vi "Mandelbrot.vi"() -> ()   [LabVIEW 2011]
doc: "This VI will create a mandelbrot fractal image. You can modify the colors by changing the map in the color map section. In addition, you can also modify the depth and color scheme by changing the iteration maximum (currently set to 50)."
uses:
  <vilib>/Utility/miscctls.llb/LVBoundsTypeDef.ctl
  <vilib>/Analysis/1siggen.llb/Ramp Pattern by Samples.vi
  <vilib>/gmath/interp.llb/Create Mesh Grid (2D) (x,y arrays).vi
  <vilib>/Analysis/NI_AALBase.lvlib
  <vilib>/gmath/NI_Gmath.lvlib
panel:
  out "Create picture name":string
  out "Zoom":dbl
  out "Min":cdb
  out "Max":cdb
  in  "Picture Folder":path
  in  "Save Button":bool
  in  "Iterations":u32=400
  in  "Resolution":u32=1000
  out "Horizontal Graduated Bar":dbl(slide)=0.999 scale=0.0..1.0
  in  "Reset":bool
  in  "Redraw":bool
  in  "stop":bool
  in  "Im_min":dbl=-2.0
  in  "Im_max":dbl=2.0
  in  "Re_min":dbl=-2.0
  in  "Re_max":dbl=2.0
  out "Intensity Graph":u32[][](graph)
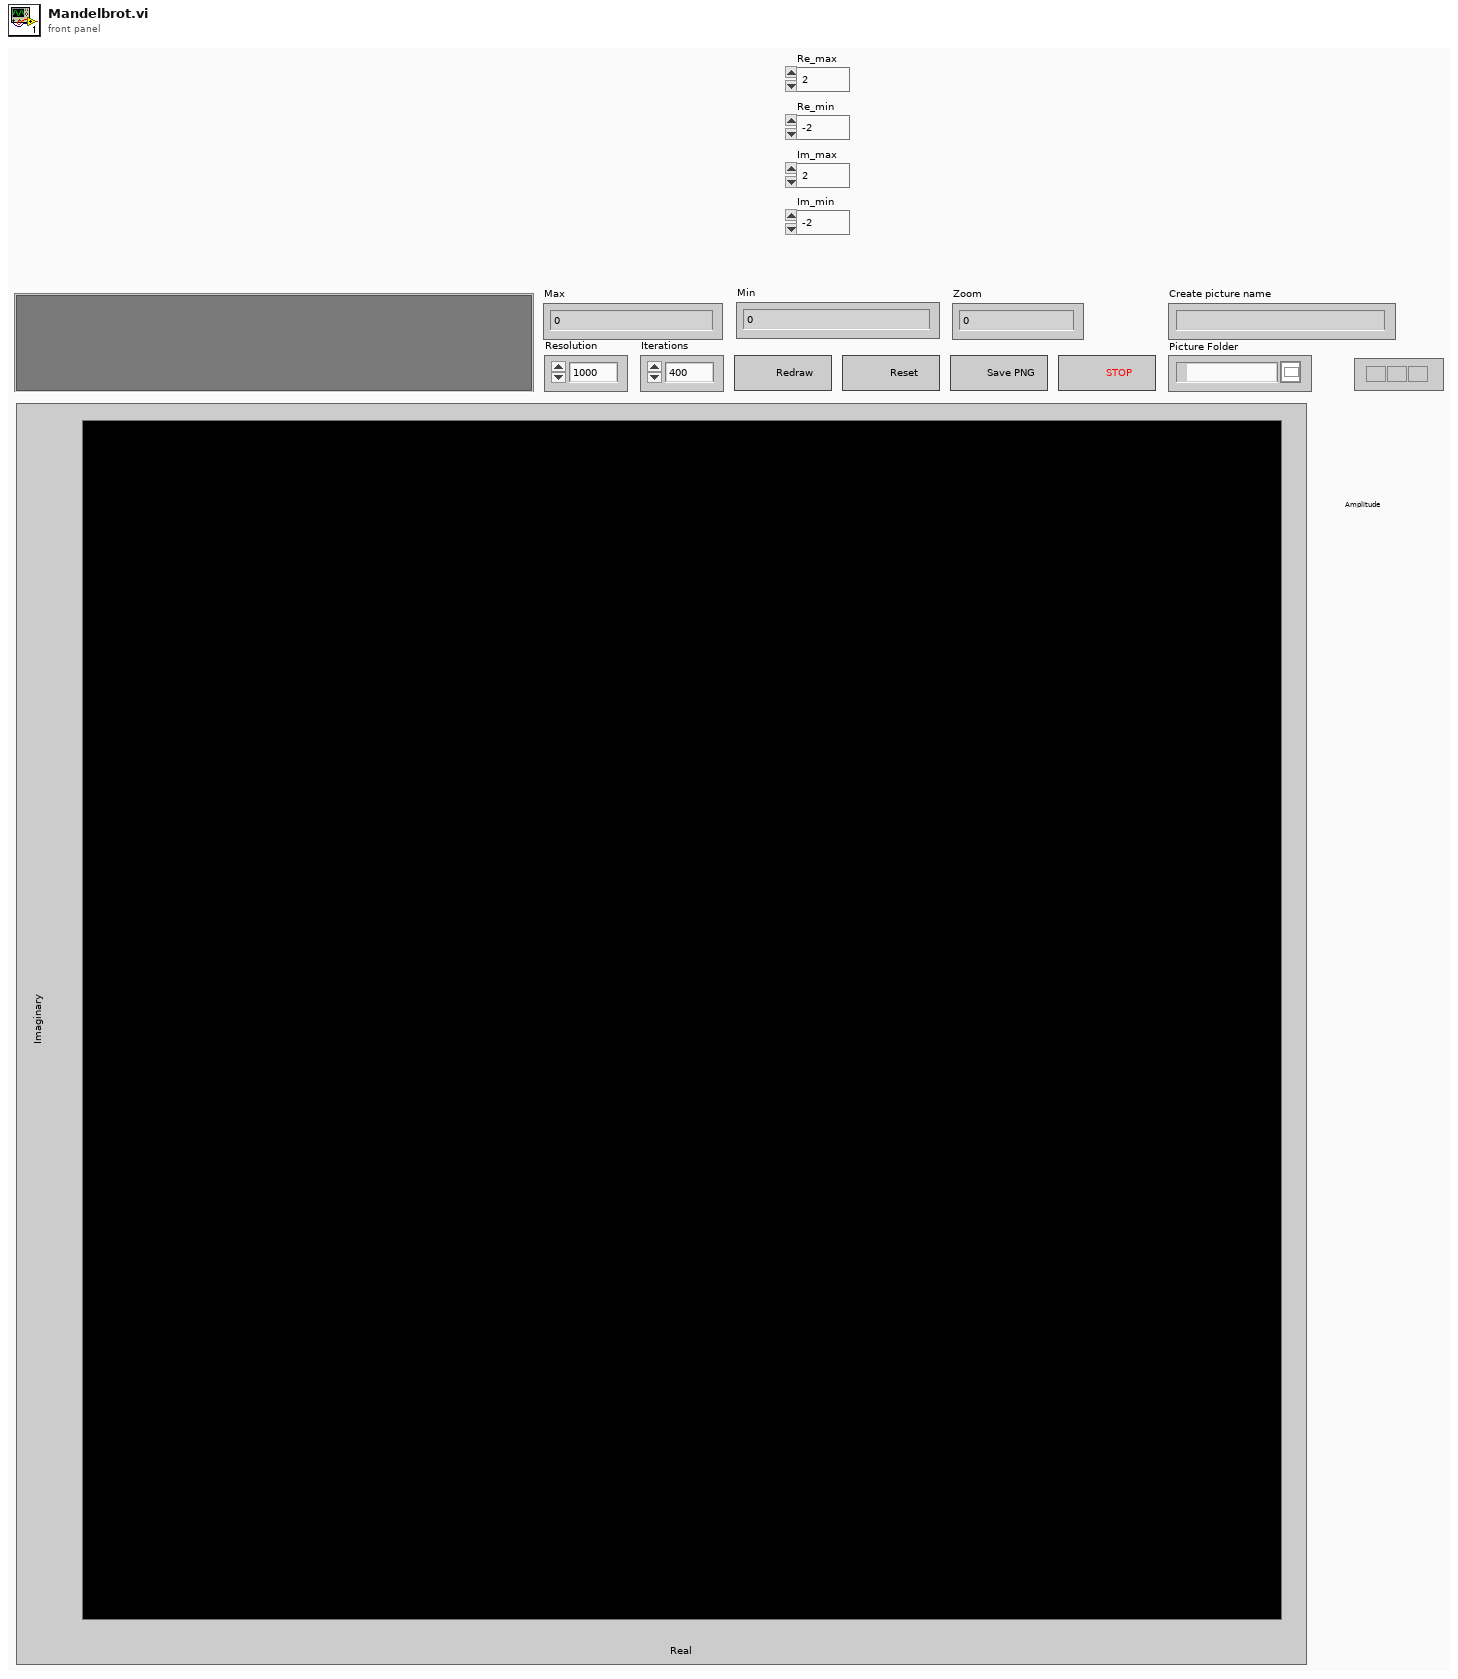
[diagram p1: front panel]
types:
  T1 = typedef "LVBoundsTypeDef.ctl" = cluster{"Width":u32, "Height":u32}
  T2 = typedef "imagedata.ctl" = cluster{"image type":i32, "image depth":i32, "image":u8[], "mask":u8[], "colors":u32[], "Rectangle":cluster{"left":i16, "top":i16, "right":i16, "bottom":i16}}
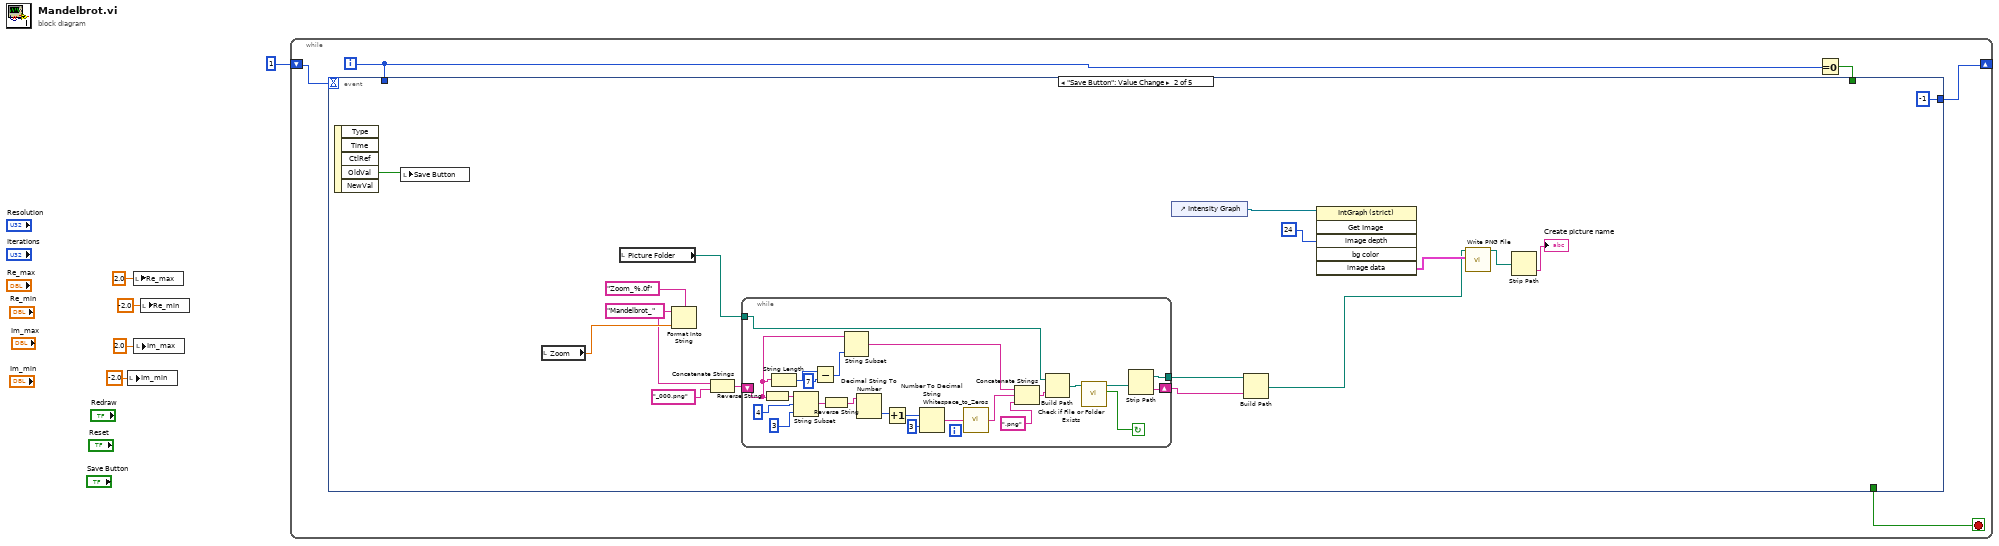
[diagram p0: block diagram]
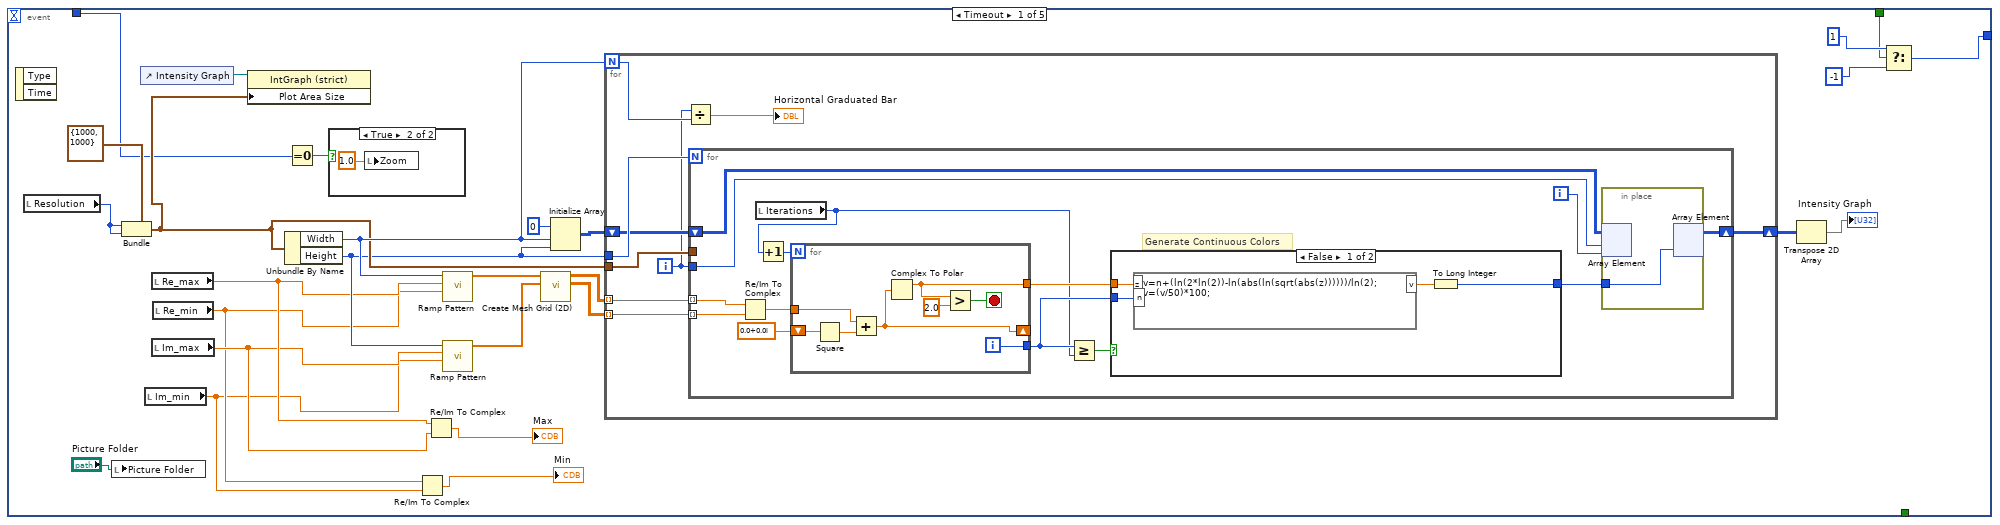
[diagram p2: hidden frame]
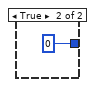
[diagram p4: hidden frame]
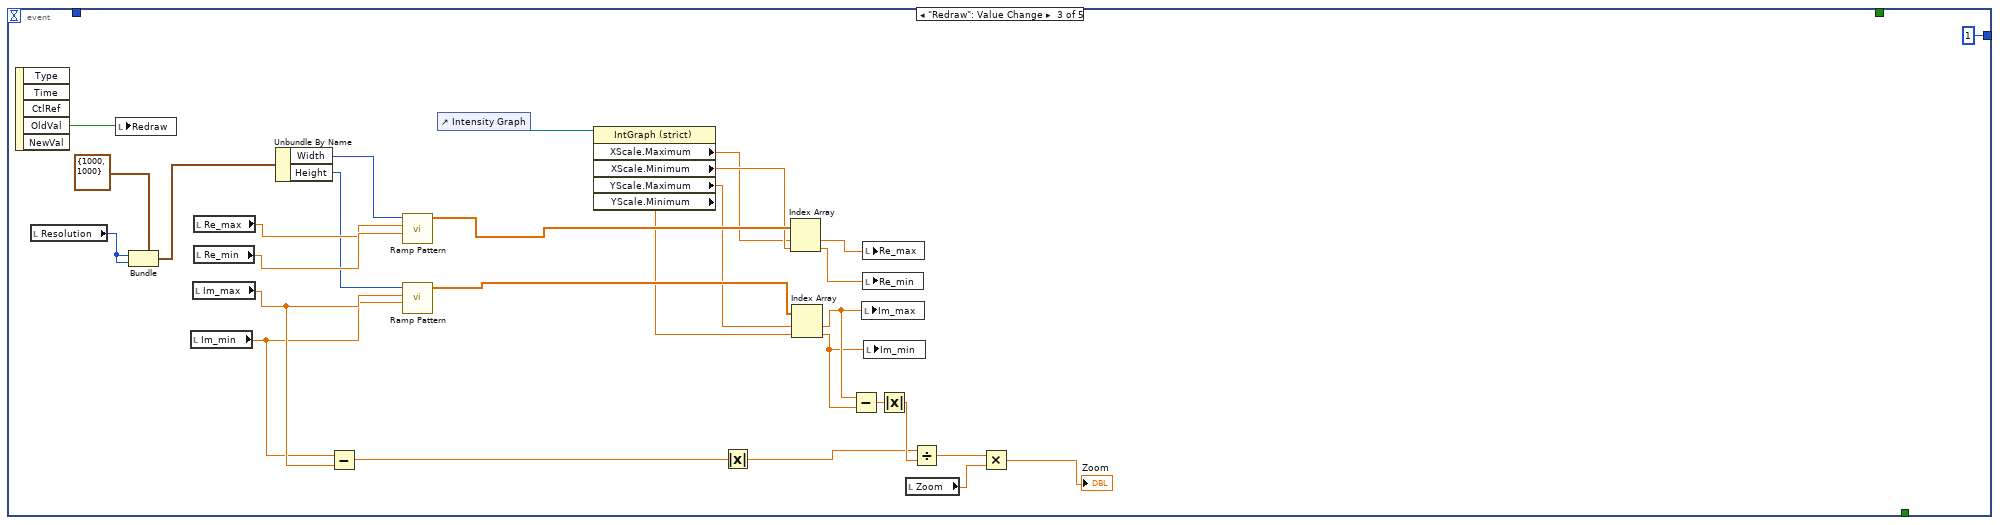
[diagram p5: hidden frame]
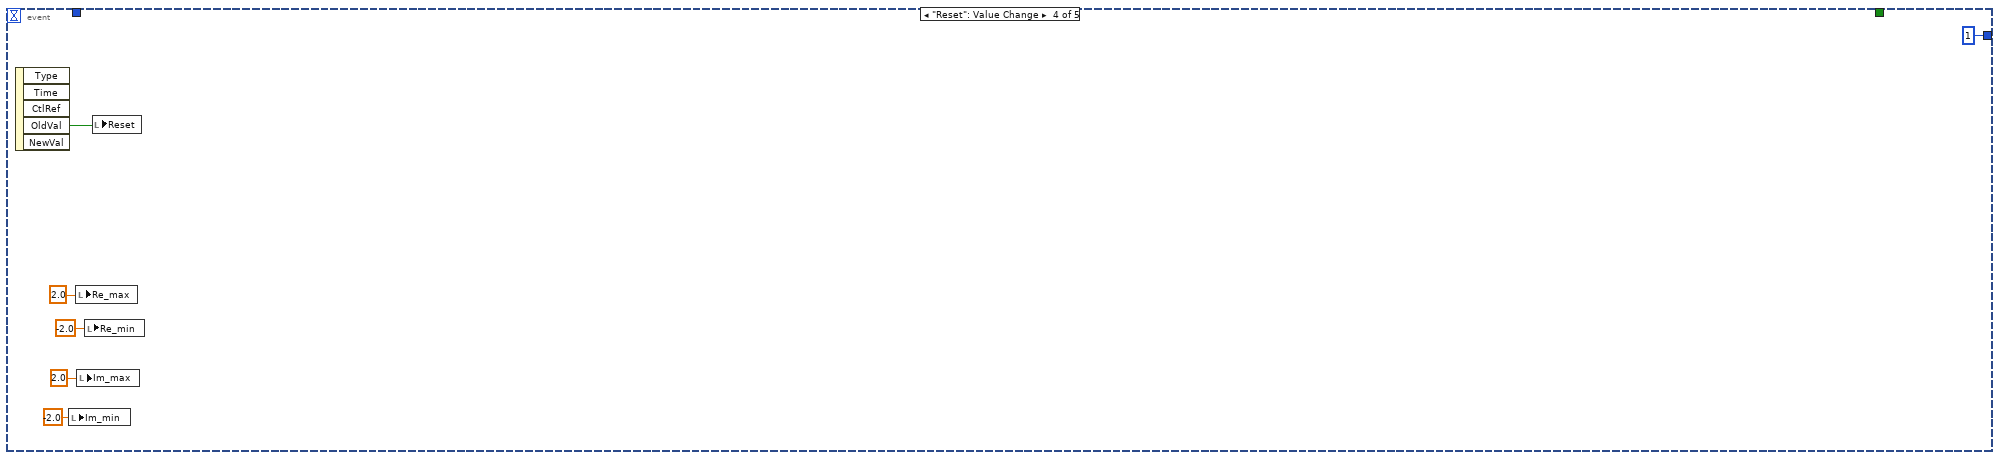
[diagram p6: hidden frame]
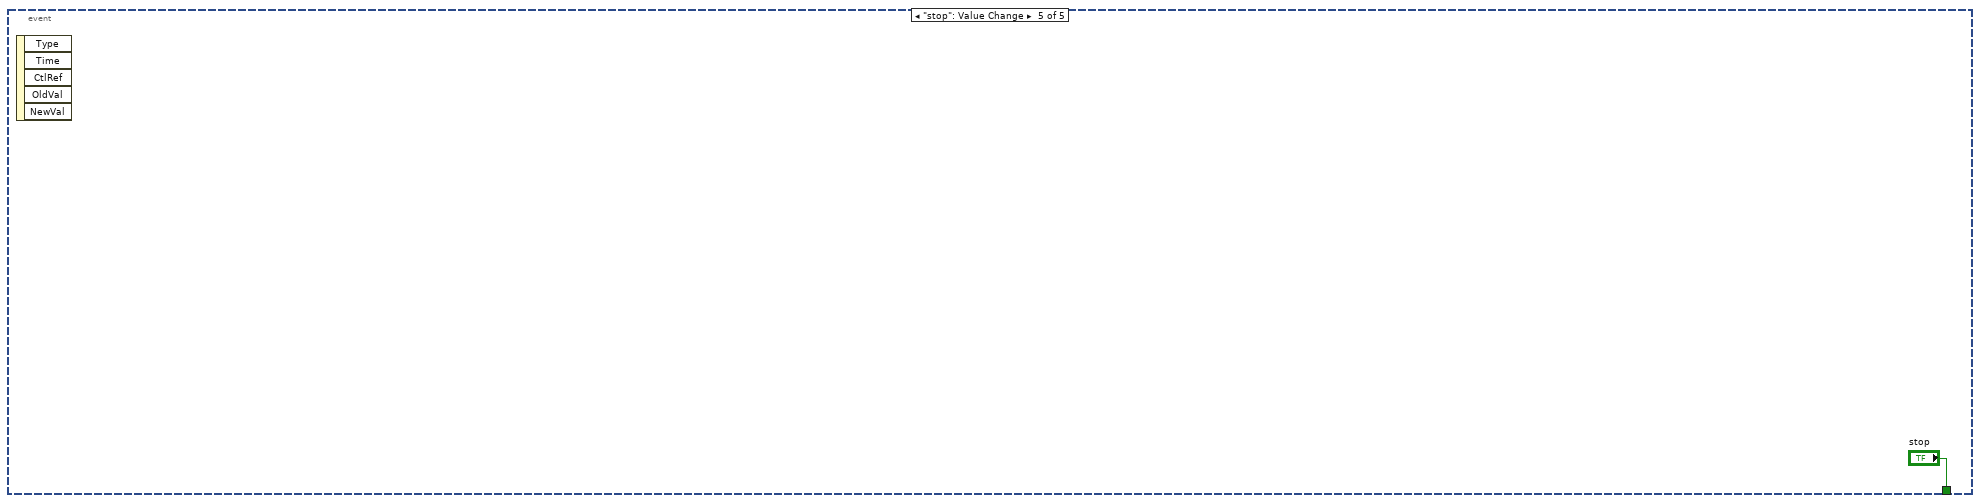
[diagram p7: hidden frame]
diagram:
  n1 = local write "Im_min"(-2.0 ("Im_min")) -> ()
  n2 = local write "Re_max"(2.0 ("Re_max")) -> ()
  n3 = local write "Im_max"(2.0 ("Im_max")) -> ()
  n4 = local write "Re_min"(-2.0 ("Re_min")) -> ()
  n5 = while {
    shift-right: [w9] -> _
    shift-left: 1 -> [w10]
    i -> [w6]
    stop <- w8 stop-if-true
    n6 = Equal To 0?(x=w6) -> (x = 0?=w7:bool)
    n7 = event shown="[1] \"Save Button\": Value Change" {
      selector: _ -> [_ _ _ _ _]
      dyn-events: _ -> [_ _ _ _ _]
      timeout: w10 -> [_ _ _ _ _]
      tunnel: [w22 -1 1 1 _] -> w9
      tunnel: [_ _ _ _ "stop"] -> w8
      tunnel: w7 -> [w23 _ _ _ _]
      tunnel: w6 -> [w13 _ _ _ _]
      event Timeout {
        n8 = event-data() -> ()  [unwired: 1 in, 2 out]
        n9 = local read "Resolution"() -> (w28:u32)
        n10 = local write "Picture Folder"("Picture Folder") -> ()
        n11 = Bundle(cluster=T1 {"Width"=1000, "Height"=1000} ("Draw Area Size"), "Width"=w28, "Height"=w28) -> (w26:T1)
        n12 = control-ref of="Intensity Graph"() -> (w27:refnum<vi>)
        n13 = local read "Im_min"() -> (w15:dbl)
        n14 = local read "Re_max"() -> (w19:dbl)
        n15 = local read "Im_max"() -> (w18:dbl)
        n16 = local read "Re_min"() -> (w16:dbl)
        n17 = property class="IntGraph (strict)"(reference=w27, "Plot Area Size"=w26) -> ()  [unwired: 1 in, 2 out]
        n18 = Unbundle By Name(w26) -> ("Width"=w34:u32, "Height"=w20:u32)
        n19 = Equal To 0?(x=w13) -> (x = 0?=w12:bool)
        n20 = case shown="True" w12 {
          frame False {
          }
          frame True {
            n21 = local write "Zoom"(1.0 ("Zoom")) -> ()
          }
        }
        n22 = Re/Im To Complex(1:w15, 2:w16) -> (0:→"Min":cdb)
        n23 = Re/Im To Complex(1:w18, 2:w19) -> (0:→"Max":cdb)
        n24 = call-poly <vilib>:"Ramp Pattern.vi"("start"=w16, "end"=w19, "samples"=w34) -> ("Ramp Pattern"=w33:dbl[])  [unwired: 7 in, 1 out]
        n25 = call-poly <vilib>:"Ramp Pattern.vi"("start"=w15, "end"=w18, "samples"=w20) -> ("Ramp Pattern"=w32:dbl[])  [unwired: 7 in, 1 out]
        n26 = call-poly <vilib>:"Create Mesh Grid (2D).vi"("y domain"=w32, "x domain"=w33) -> ("Y"=w30:dbl[][], "X"=w31:dbl[][])  [unwired: 7 in, 1 out]
        n27 = Initialize Array(u32 0 ("element"), w34, w20) -> (w36:u32[][])
        n28 = for {
          N: w34 -> [w41]
          tunnel: w20 -> [w47]
          tunnel: w26 -> [w46]
          shift-right: [w44] -> w35
          shift-left: w36 -> [w45]
          tunnel: w31 -> [w43] mode=indexing
          tunnel: w30 -> [w42] mode=indexing
          i -> [w40]
          n29 = Divide(x=w40, y=w41) -> (x/y=→"Horizontal Graduated Bar":dbl)
          n30 = for {
            N: w47 -> [_]
            tunnel: w40 -> [w56]
            tunnel: w46 -> [_]
            shift-right: [w57] -> w44
            shift-left: w45 -> [w58]
            tunnel: w43 -> [w51] mode=indexing
            tunnel: w42 -> [w50] mode=indexing
            i -> [w55]
            # "Generate Continuous Colors"
            n31 = Re/Im To Complex(1:w50, 2:w51) -> (0:w52:cdb)
            n32 = local read "Iterations"() -> (w49:u32)
            n33 = Increment(x=w49) -> (x+1=w48:u32)
            n34 = for {
              N: w48 -> [_]
              tunnel: w52 -> [w68]
              shift-right: [w66] -> _
              shift-left: cdb 0.0+0.0i ("x + iy") -> [w69]
              tunnel: [w63] -> w60
              tunnel: [w62] -> w59
              i -> [w62]
              stop <- w64 stop-if-true
              n35 = Square(x=w69) -> (x^2=w67:cdb)
              n36 = Add(x=w68, y=w67) -> (x+y=w66:cdb)
              n37 = Complex To Polar(r * e^(i*theta)=w66) -> (r=w63:dbl)  [unwired: 1 out]
              n38 = Greater?(x=w63, y=2.0) -> (0:w64:bool)
            }
            n39 = Greater Or Equal?(x=w59, y=w49) -> (x >= y?=w61:bool)
            n40 = case shown="False" w61 {
              tunnel: [w74 0] -> w54
              tunnel: w60 -> [w73 _]
              tunnel: w59 -> [w72 _]
              frame False {
                n41 = formula code="v=n+(ln(2*ln(2))-ln(abs(ln(sqrt(abs(z))))))/ln(2);\nv=(v/50)*100;"("z"=w73, "n"=w72) -> ("v"=w71:dbl)
                n42 = To Long Integer(number=w71) -> (32bit integer=w74:i32)
              }
              frame True {
              }
            }
            n43 = in-place {
              in-place-border: w54 -> [w70]
              n44 = in-place-array #1(w58, w56, w55) -> ()  [unwired: 1 out]
              n45 = in-place-array #1(w70) -> (w57:u32[][])  [unwired: 2 out]
            }
          }
        }
        n46 = Transpose 2D Array(2D array=w35) -> (transposed array=→"Intensity Graph":u32[][])
        n47 = Select(t=1, s=w23, f=-1) -> (s? t:f=w22:i32)
      }
      event "Save Button": Value Change {
        n48 = event-data() -> ("OldVal"=w92:bool)  [unwired: 1 in, 4 out]
        n49 = local write "Save Button"(w92) -> ()
        n50 = local read "Zoom"() -> (w85:dbl)
        n51 = local read "Picture Folder"() -> (w84:path)
        n52 = Format Into String(format string="Zoom_%.0f", initial string="Mandelbrot_", w85) -> (resulting string=w78:string)  [unwired: 1 in, 1 out]
        n53 = Concatenate Strings(w78, "_000.png" ("string")) -> (w79:string)
        n54 = while {
          shift-right: [w110] -> w76
          shift-left: w79 -> [w101]
          tunnel: w84 -> [w115]
          tunnel: [w109] -> w83
          stop <- w113 continue-if-true
          n55 = Reverse String(1:w101) -> (0:w108:string)
          n56 = String Length(string=w101) -> (length=w100:i32)
          n57 = String Subset(string=w108, offset (0)=4, length (rest)=3 ("length (rest)")) -> (substring=w106:string)
          n58 = Subtract(x=w100, y=7) -> (x-y=w98:i32)
          n59 = Reverse String(1:w106) -> (0:w105:string)
          n60 = String Subset(string=w101, length (rest)=w98) -> (substring=w97:string)  [unwired: 1 in]
          n61 = Decimal String To Number(string=w105) -> (number=w104:i32)  [unwired: 2 in, 1 out]
          n62 = Increment(x=w104) -> (x+1=w103:i32)
          n63 = Number To Decimal String(number=w103, width (-)=i16 3) -> (decimal integer string=w96:string)
          n64 = call "Whitespace_to_Zeros.vi"("Input String"=w96) -> ("Output String"=w95:string)  [unwired: 6 in]
          n65 = Concatenate Strings(w97, w95, ".png" ("string")) -> (w112:string)
          n66 = Build Path(base path=w115, name or relative path=w112) -> (appended path=w114:path)
          n67 = call <vilib>:"Check if File or Folder Exists.vi"("path"=w114) -> ("file or folder exists?"=w113:bool, "dup path"=w111:path)  [unwired: 8 in, 1 out]
          n68 = Strip Path(path=w111) -> (stripped path=w109:path, name=w110:string)
        }
        n69 = control-ref of="Intensity Graph"() -> (w91:refnum<vi>)
        n70 = Build Path(base path=w83, name or relative path=w76) -> (appended path=w82:path)
        n71 = invoke class="IntGraph (strict)" method="Get Image"(reference=w91, "image depth"=24 ("Image Depth")) -> ("image data"=w89:T2)  [unwired: 4 in, 5 out]
        n72 = call <vilib>:"Write PNG File.vi"("image data"=w89, "path to PNG file"=w82) -> ("path"=w81:path)  [unwired: 8 in, 1 out]
        n73 = Strip Path(path=w81) -> (name=→"Create picture name":string)  [unwired: 1 out]
      }
      event "Redraw": Value Change {
        n74 = event-data() -> ("OldVal"=w144:bool)  [unwired: 1 in, 4 out]
        n75 = local read "Resolution"() -> (w128:u32)
        n76 = local write "Redraw"(w144) -> ()
        n77 = Bundle(cluster=T1 {"Width"=1000, "Height"=1000} ("Draw Area Size"), "Width"=w128, "Height"=w128) -> (w127:T1)
        n78 = local read "Im_min"() -> (w125:dbl)
        n79 = local read "Im_max"() -> (w126:dbl)
        n80 = local read "Re_max"() -> (w141:dbl)
        n81 = local read "Re_min"() -> (w142:dbl)
        n82 = Unbundle By Name(w127) -> ("Width"=w139:u32, "Height"=w140:u32)
        n83 = Subtract(x=w125, y=w126) -> (x-y=w120:dbl)
        n84 = call-poly <vilib>:"Ramp Pattern.vi"("start"=w142, "end"=w141, "samples"=w139) -> ("Ramp Pattern"=w137:dbl[])  [unwired: 7 in, 1 out]
        n85 = call-poly <vilib>:"Ramp Pattern.vi"("start"=w125, "end"=w126, "samples"=w140) -> ("Ramp Pattern"=w133:dbl[])  [unwired: 7 in, 1 out]
        n86 = control-ref of="Intensity Graph"() -> (w138:refnum<vi>)
        n87 = property class="IntGraph (strict)"(reference=w138) -> ("XScale.Maximum"=w130:dbl, "XScale.Minimum"=w135:dbl, "YScale.Maximum"=w132:dbl, "YScale.Minimum"=w131:dbl)  [unwired: 1 in, 2 out]
        n88 = Absolute Value(x=w120) -> (abs(x)=w118:dbl)
        n89 = Index Array(array=w137, index #1=w130, index #2=w135) -> (element #1=w136:dbl, element #2=w134:dbl)
        n90 = Index Array(array=w133, index #1=w132, index #2=w131) -> (element #1=w124:dbl, element #2=w123:dbl)
        n91 = Subtract(x=w124, y=w123) -> (x-y=w121:dbl)
        n92 = local write "Im_max"(w124) -> ()
        n93 = local write "Re_max"(w136) -> ()
        n94 = local write "Re_min"(w134) -> ()
        n95 = local write "Im_min"(w123) -> ()
        n96 = Absolute Value(x=w121) -> (abs(x)=w119:dbl)
        n97 = local read "Zoom"() -> (w116:dbl)
        n98 = Divide(x=w118, y=w119) -> (x/y=w122:dbl)
        n99 = Multiply(x=w122, y=w116) -> (x*y=→"Zoom":dbl)
      }
      event "Reset": Value Change {
        n100 = event-data() -> ("OldVal"=w150:bool)  [unwired: 1 in, 4 out]
        n101 = local write "Im_min"(-2.0 ("Im_min")) -> ()
        n102 = local write "Re_max"(2.0 ("Re_max")) -> ()
        n103 = local write "Im_max"(2.0 ("Im_max")) -> ()
        n104 = local write "Re_min"(-2.0 ("Re_min")) -> ()
        n105 = local write "Reset"(w150) -> ()
      }
      event "stop": Value Change {
        n106 = event-data() -> ()  [unwired: 1 in, 5 out]
      }
    }
  }
